vi "Init Task.vi"(4 "counter":tag, 6 "line grouping":i32(ring) items=["one channel for each line", "one channel for all lines"], 7 "physical channels":tag, 8 "error in (no error)":errorcluster, 9 "name":string, 10 "DAQmxTaksContainer_General IN":refnum<class "DAQmxTaksContainer_General.lvclass">, 11 "DAQmxTaskDOutput in":refnum<class "DAQmxTaskDOutput.lvclass">) -> (0 "error out":errorcluster, 3 "DAQmxTaskDOutput out":refnum<class "DAQmxTaskDOutput.lvclass">)   [LabVIEW 2015, in "DAQmxTaskDOutput.lvclass"]
uses:
  DAQmxTaskDOutput.lvclass
  DAQmxTaskContainer_General/DAQmxTaksContainer_General.lvclass
  DAQmxTask.lvclass/DAQmxTask.ctl
  <vilib>/DAQmx/create/channels.llb/DAQmx Create Channel (DO-Digital Output).vi
  DAQmxTask.lvclass
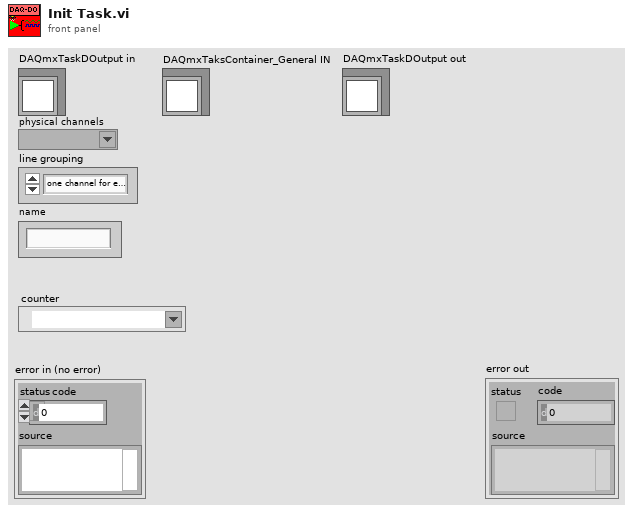
[diagram p1: front panel]
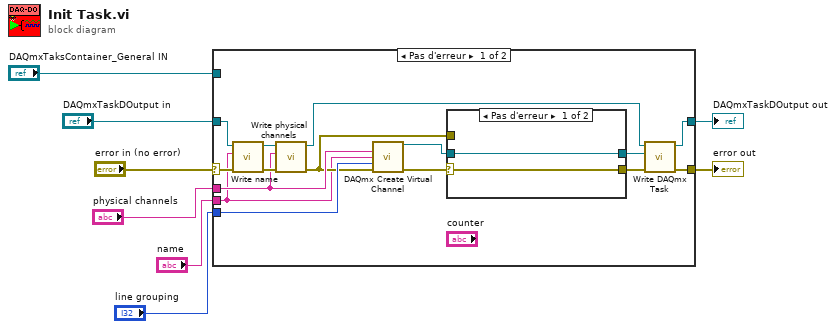
[diagram p0: block diagram]
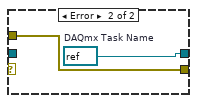
[diagram p2: hidden frame]
diagram:
  n1 = case shown="Pas d'erreur" "error in (no error)" {
    selector: "error in (no error)" -> [w22 w29]
    tunnel: "DAQmxTaskDOutput in" -> [w23 w28]
    tunnel: "name" -> [w11 _]
    tunnel: "physical channels" -> [w18 _]
    tunnel: "line grouping" -> [w17 _]
    tunnel: [w9 w29] -> w3
    tunnel: "DAQmxTaksContainer_General IN" -> [_ _]
    tunnel: [w10 w28] -> w1
    frame No Error {
      n2 = call "Write name.vi"("error in (no error)"=w22, "name"=w11, "DAQmxTask in"=w23) -> ("error out"=w20:errorcluster, "DAQmxTask out"=w21:refnum<class "DAQmxTaskDOutput.lvclass">)  [unwired: 7 in]
      n3 = call "Write physical channels.vi"("error in (no error)"=w20, "physical channels"=w18, "DAQmxTask in"=w21) -> ("error out"=w14:errorcluster, "DAQmxTask out"=w19:refnum<class "DAQmxTaskDOutput.lvclass">)  [unwired: 7 in]
      n4 = call-poly <vilib>:"DAQmx Create Virtual Channel.vi"("lines"=w18, "name to assign"=w11, "line grouping"=w17, "error in"=w14) -> ("task out"=w12:refnum<k21>, "error out"=w13:errorcluster)  [unwired: 10 in]
      n5 = case shown="Pas d'erreur" w13 {
        selector: w13 -> [w24 _]
        tunnel: [w25 w26] -> w15
        tunnel: w12 -> [w25 _]
        tunnel: [w24 w27] -> w16
        tunnel: w14 -> [_ w27]
        frame No Error {
        }
        frame Error {
          w26 = refnum<k21> refnum  # DAQmx Task Name
        }
      }
      n6 = call "Write DAQmx Task.vi"("error in (no error)"=w16, "DAQmx Task Name"=w15, "DAQmxTask in"=w19) -> ("error out"=w9:errorcluster, "DAQmxTask out"=w10:refnum<class "DAQmxTaskDOutput.lvclass">)  [unwired: 7 in]
    }
    frame Error {
    }
  }
  "error out" <- w3
  "DAQmxTaskDOutput out" <- w1
